vi "SendMultipleUserEventMessages.vi"(8 "error in":errorcluster, 9 "message data []":variant[](array[variant]), 10 "message names []":string[](array[string]), 11 "message ref in":refnum<class "CLM_LocalMessage_UserEvent.lvclass">) -> (0 "error out":errorcluster, 3 "message ref out":refnum<class "CLM_LocalMessage_UserEvent.lvclass">)   [LabVIEW 2013, in "CLM_LocalMessage_UserEvent.lvclass"]
uses:
  CLM_LocalMessage_UserEvent.lvclass
  CLM_LocalMessage_UserEvent.lvclass/CLM_LocalMessage_UserEvent.ctl
  LocalMessage/BundleMessageCluster.vi
  SendUserEventMessage_Cluster.vi
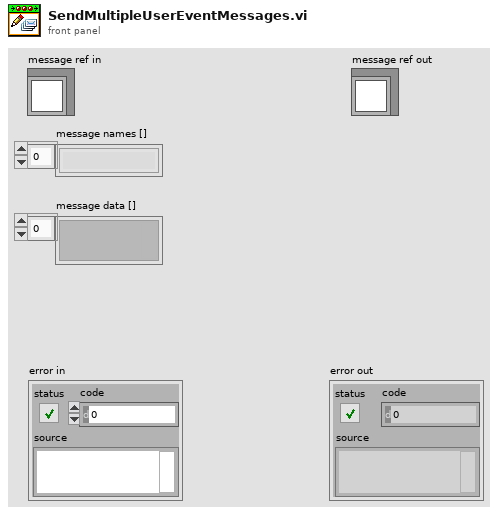
[diagram p1: front panel]
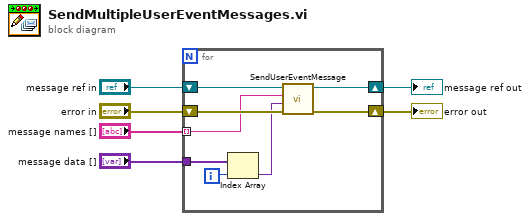
[diagram p0: block diagram]
diagram:
  n1 = for {
    shift-right: [w12] -> w1
    shift-left: "error in" -> [w14]
    shift-right: [w13] -> w2
    shift-left: "message ref in" -> [w7]
    tunnel: "message names []" -> [w11] mode=indexing
    tunnel: "message data []" -> [w10]
    i -> [w9]
    n2 = Index Array(array=w10, index=w9) -> (element=w8:variant)
    n3 = call "SendUserEventMessage.vi"("error in"=w14, "data"=w8, "name"=w11, "message ref in"=w7) -> ("error out"=w12:errorcluster, "message ref out"=w13:refnum<class "CLM_LocalMessage_UserEvent.lvclass">)  [unwired: 6 in]
  }
  "error out" <- w1
  "message ref out" <- w2
